vi "Configure Multi Eval Meas List Segment Subcarrier Spacing.vi"(7 "Subcarrier Spacing (30 kHz)":i32(ring)=1 items=["15 kHz", "30 kHz", "60 kHz"], 8 "error in (no error)":errorcluster, 9 "Segment (1)":i32=1, 10 "Instance (1)":T1=1, 11 "VISA resource name":refnum<visa-resource-name>) -> (0 "error out":errorcluster, 3 "VISA resource name out":refnum<visa-resource-name>)   [LabVIEW 2020, in "Rohde&Schwarz CMWXP NR FR1 Measurement.lvlib"]
doc: "Selects the subcarrier spacing used in segment <no>, for all carriers.\n\nAttribute:\nRSCMWXPNRFR1M_ATTR_MULTI_EVAL_MEAS_LIST_SEGMENT_SUBCARRIER_SPACING\n\nRemote-control command:\nCONFigure:NRSub:MEAS<i>:LIST:SEGMent<no>:CCALl:TXBWidth:SCSPacing"
uses:
  <instrlib>/Rohde&Schwarz CMWXP NR FR1 Measurement/Rohde&Schwarz CMWXP NR FR1 Measurement.lvlib
  <instrlib>/Rohde&Schwarz CMWXP NR FR1 Measurement/Private/_Instance.ctl
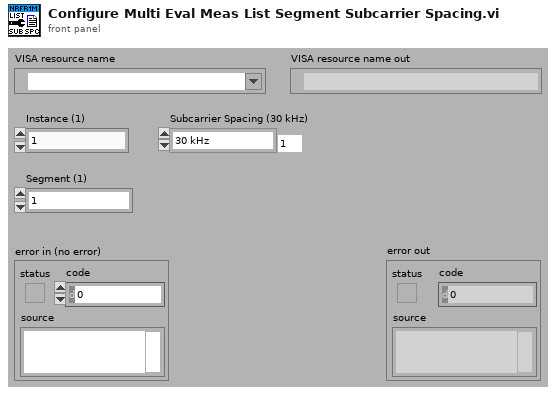
[diagram p1: front panel]
types:
  T1 = typedef "Rohde&Schwarz CMWXP NR FR1 Measurement.lvlib/_Instance.ctl" = i32
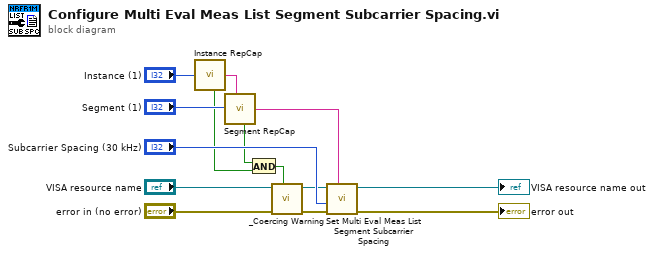
[diagram p0: block diagram]
diagram:
  n1 = call <instrlib>:"Instance RepCap.vi"("Instance In"="Instance (1)") -> ("In Range?"=w2:bool, "RepCap Identifier Out"=w9:string)  [unwired: 1 in]
  n2 = call <instrlib>:"Segment RepCap.vi"("Segment In"="Segment (1)", "RepCap String In (\"\")"=w9) -> ("In Range?"=w1:bool, "RepCap Identifier Out"=w8:string)
  n3 = And(x=w1, y=w2) -> (x .and. y?=w3:bool)
  n4 = call <instrlib>:"_Coercing Warning.vi"("In Range?"=w3, "error in (no error)"="error in (no error)", "VISA resource name"="VISA resource name") -> ("error out"=w5:errorcluster, "VISA resource name out"=w4:refnum<visa-resource-name>)  [unwired: 7 in]
  n5 = call "Set Multi Eval Meas List Segment Subcarrier Spacing"("Repeated Capabilities"=w8, "error in (no error)"=w5, "Multi Eval Meas List Segment Subcarrier Spacing (0 - 15 kHz)"="Subcarrier Spacing (30 kHz)", "instrument handle"=w4) -> ("error out"=→"error out":errorcluster, "instrument handle out"=→"VISA resource name out":refnum<visa-resource-name>)  [unwired: 6 in]
